vi "OUT_24_BIT.vi"(8 "Array":bool[](array[boolean]), 9 "error in":errorcluster, 11 "String":string) -> (0 "error out":errorcluster)   [LabVIEW 2017]
uses:
  <vilib>/DAQmx/write.llb/DAQmx Write (Digital 1D Bool 1Chan 1Samp).vi
  <vilib>/DAQmx/create/channels.llb/DAQmx Create Channel (DO-Digital Output).vi
  <vilib>/DAQmx/miscellaneous.llb/DAQmx Fill In Error Info.vi
panel:
  in  "lines":tag
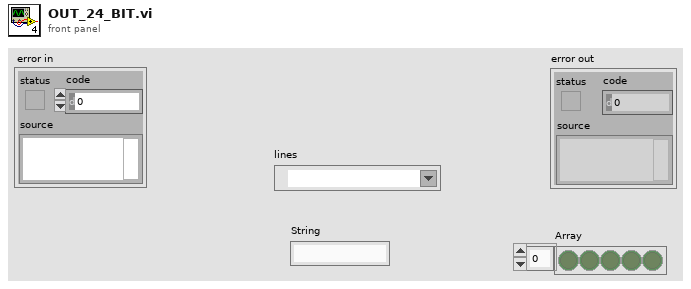
[diagram p1: front panel]
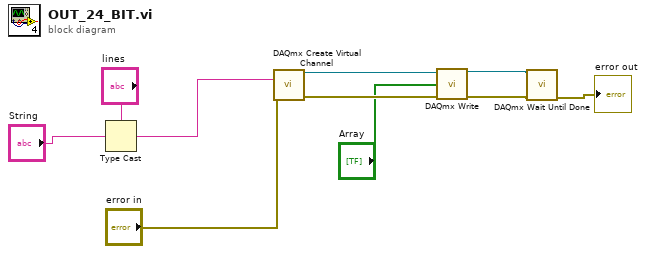
[diagram p0: block diagram]
diagram:
  n1 = Type Cast(type="lines", x="String") -> (*(type *) &x=w6:tag)
  n2 = call-poly <vilib>:"DAQmx Create Virtual Channel.vi"("lines"=w6, "error in"="error in") -> ("task out"=w10:refnum<k21>, "error out"=w9:errorcluster)  [unwired: 12 in]
  n3 = call-poly <vilib>:"DAQmx Write.vi"("task/channels in"=w10, "data"="Array", "error in"=w9) -> ("task out"=w5:refnum<k21>, "error out"=w4:errorcluster)  [unwired: 10 in, 1 out]
  n4 = call <vilib>:"DAQmx Wait Until Done.vi"("task/channels in"=w5, "error in"=w4) -> ("error out"=→"error out":errorcluster)  [unwired: 12 in, 1 out]
